vi "Read_FPGA_FIFOs.vi"(6 "TargetB":T1=enum."4", 7 "TargetA":T1, 8 "error in":errorcluster, 9 "#Elements":u32, 11 "FPGA VI Ref":refnum<k20>) -> (0 "error out":errorcluster, 1 "Elements Remaining":u32, 2 "AcqDataB":T2, 3 "AcqDataA":T2)   [LabVIEW 2018]
uses:
  Controls/Clusts/AcqData.ctl
  Controls/Enums/TargetNumber.ctl
  Controls/Clusts/SaturationMonitor.ctl
  Controls/Clusts/FromFPGA_Clust.ctl
  <vilib>/Analysis/baseanly.llb/Mean (DBL).vi
  <vilib>/Utility/error.llb/Error Cluster From Error Code.vi
  <vilib>/rvi/errors/niLvFpgaAdjustHostInterfaceError.vi
  <vilib>/rvi/interface/nirviReadWriteControl/nirviReadWriteControl.xnode
  <vilib>/rvi/interface/nirviMethod/nirviMethod.xnode
  <vilib>/FPGAPlugInAG/Dynamic/niLvFpga_ReadFifo_Dynamic.vi
  <vilib>/rvi/errors/niLvFpgaMergeErrorWithErrorCode.vi
  <vilib>/Analysis/NI_AALBase.lvlib
  NiFpgaLv.dll
  <vilib>/rvi/interface/Simulation/niFpgaSimulationCallBeginRW.vi
panel:
  out "Data":fxp<+/-,24,1>[](array[numeric])
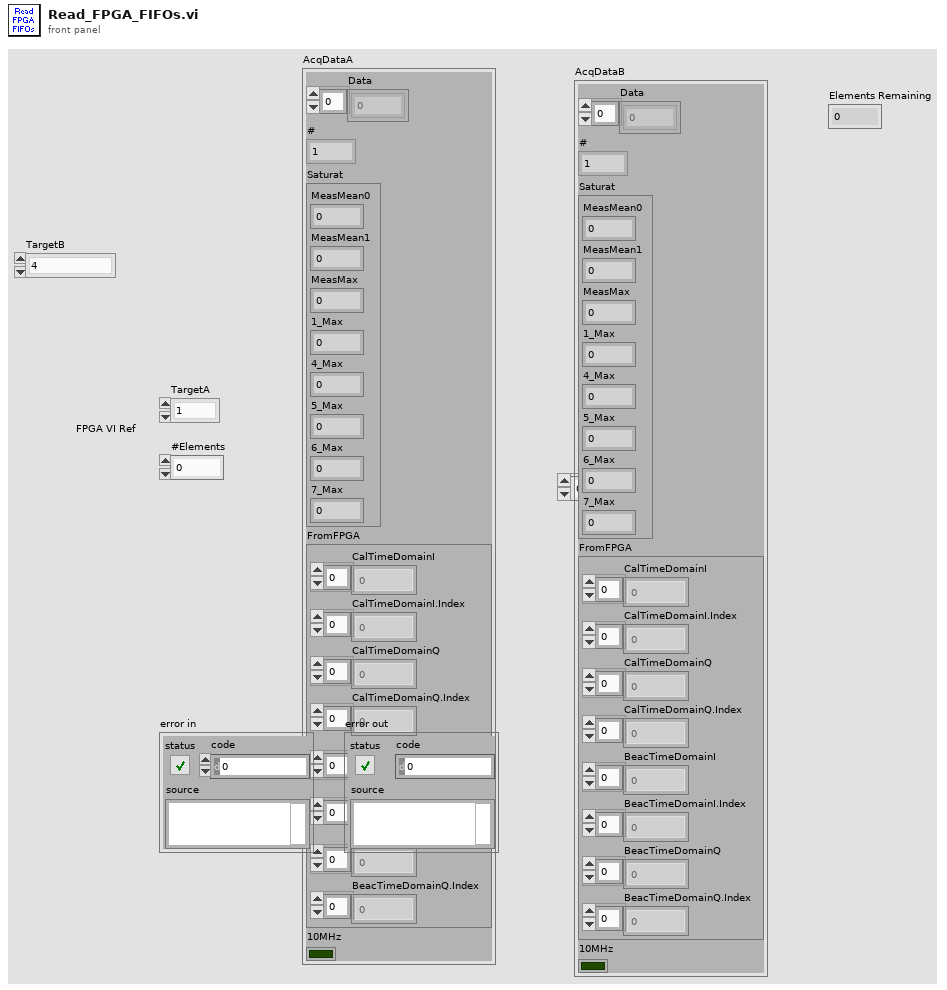
[diagram p1: front panel]
types:
  T1 = typedef "TargetNumber.ctl" = enum16{"1", "2", "3", "4"}
  T2 = typedef "AcqData.ctl" = cluster{"Data":fxp<+/-,24,1>[], "#":T1, "Saturat":T3, "FromFPGA":T4, "10MHz":bool}
  T3 = typedef "SaturationMonitor.ctl" = cluster{"MeasMean0":dbl, "MeasMean1":dbl, "MeasMax":dbl, "1_Max":dbl, "4_Max":dbl, "5_Max":dbl, "6_Max":dbl, "7_Max":dbl}
  T4 = typedef "FromFPGA_Clust.ctl" = cluster{"CalTimeDomainI":ext[], "CalTimeDomainI.Index":ext[], "CalTimeDomainQ":ext[], "CalTimeDomainQ.Index":ext[], "BeacTimeDomainI":ext[], "BeacTimeDomainI.Index":ext[], "BeacTimeDomainQ":ext[], "BeacTimeDomainQ.Index":ext[]}
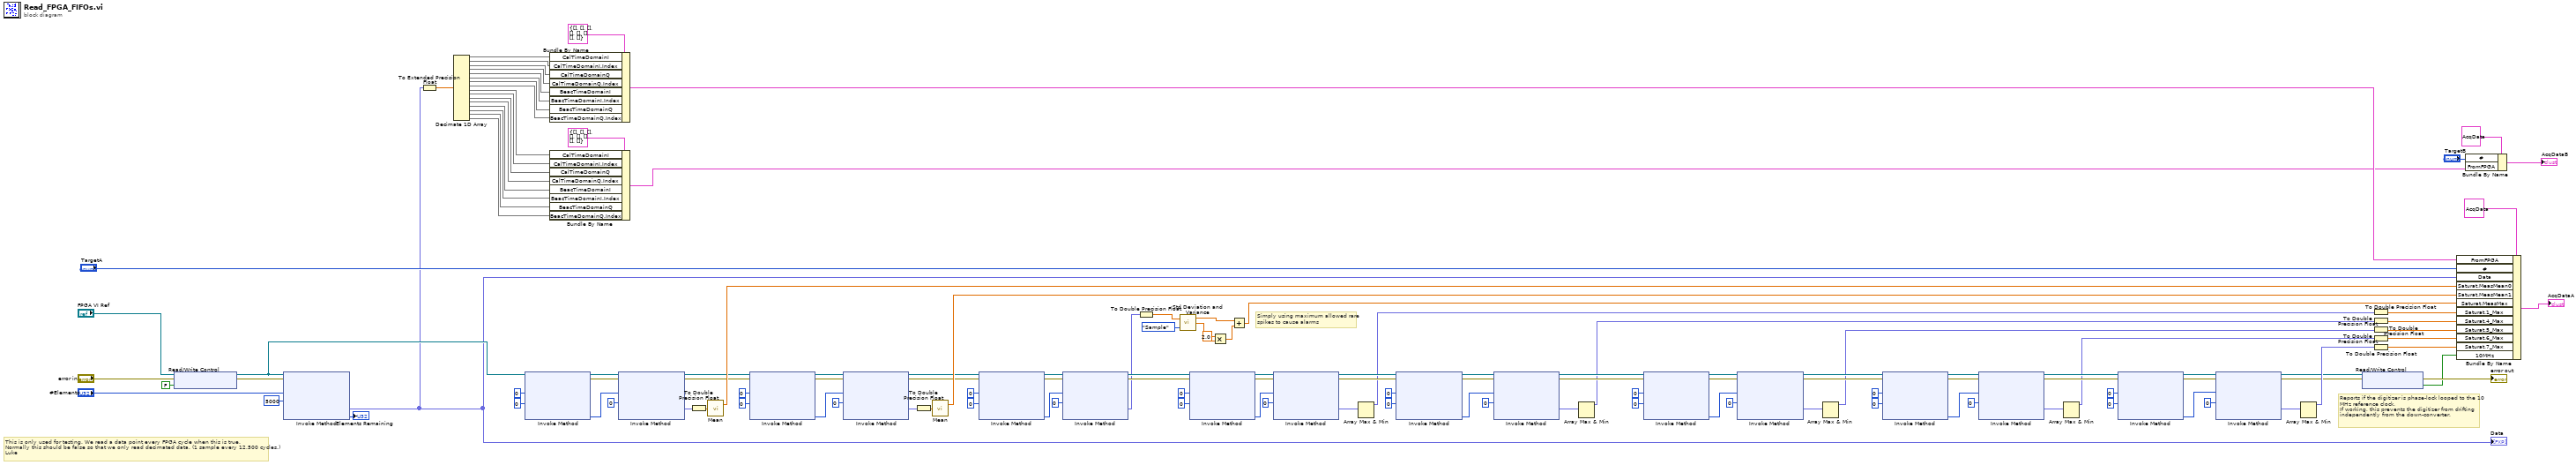
[diagram p0: block diagram]
diagram:
  # "Simply using maximum allowed rare\nspikes to cause alarms"
  # "Reports if the digitizer is phase-lock looped to the 10 MHz reference clock.\nIf working, this prevents the digitizer from drifting independently from the down-converter."
  # "This is only used for testing. We read a data point every FPGA cycle when this is true.\nNormally this should be false so that we only read decimated data. (1 sample every 12,500 cycles.)\nLuke"
  n1 = xnode "Read/Write Control"("FPGA VI Reference In"="FPGA VI Ref", "error in"="error in", "AllData_EvenInvalid"=FALSE ("EnableFIFO")) -> ("FPGA VI Reference Out"=w40:refnum<k20>, "error out"=w41:errorcluster)
  n2 = xnode "Invoke Method"("FPGA VI Reference In"=w40, "error in"=w41, "Number of Elements"="#Elements", "Timeout (ms)"=5000) -> ("Data"=w33:fxp<+/-,24,1>[], "Elements Remaining"=→"Elements Remaining":u32)  [unwired: 2 out]
  "Data" <- w33
  n3 = To Extended Precision Float(1:w33) -> (0:w30:ext[])
  n4 = Decimate 1D Array(w30) -> (w31:ext[], w29:ext[], w28:ext[], w27:ext[], w26:ext[], w25:ext[], w24:ext[], w23:ext[], w22:ext[], w21:ext[], w20:ext[], w19:ext[], w18:ext[], w17:ext[], w16:ext[], w15:ext[])
  n5 = xnode "Invoke Method"("FPGA VI Reference In"=w40, "Number of Elements"=u32 0, "Timeout (ms)"=0) -> ("FPGA VI Reference Out"=w115:refnum<k20>, "error out"=w111:errorcluster, "Elements Remaining"=w112:u32)  [unwired: 1 in, 1 out]
  n6 = Bundle By Name(cluster=T4 {"CalTimeDomainI"=[], "CalTimeDomainI.Index"=[], "CalTimeDomainQ"=[], "CalTimeDomainQ.Index"=[], "BeacTimeDomainI"=[], "BeacTimeDomainI.Index"=[], "BeacTimeDomainQ"=[], "BeacTimeDomainQ.Index"=[]} ("FromFPGA"), "CalTimeDomainI"=w31, "CalTimeDomainI.Index"=w29, "CalTimeDomainQ"=w28, "CalTimeDomainQ.Index"=w27, "BeacTimeDomainI"=w26, "BeacTimeDomainI.Index"=w25, "BeacTimeDomainQ"=w24, "BeacTimeDomainQ.Index"=w23) -> (w14:T4)
  n7 = Bundle By Name(cluster=T4 {"CalTimeDomainI"=[], "CalTimeDomainI.Index"=[], "CalTimeDomainQ"=[], "CalTimeDomainQ.Index"=[], "BeacTimeDomainI"=[], "BeacTimeDomainI.Index"=[], "BeacTimeDomainQ"=[], "BeacTimeDomainQ.Index"=[]} ("FromFPGA"), "CalTimeDomainI"=w22, "CalTimeDomainI.Index"=w21, "CalTimeDomainQ"=w20, "CalTimeDomainQ.Index"=w19, "BeacTimeDomainI"=w18, "BeacTimeDomainI.Index"=w17, "BeacTimeDomainQ"=w16, "BeacTimeDomainQ.Index"=w15) -> (w13:T4)
  n8 = xnode "Invoke Method"("FPGA VI Reference In"=w115, "error in"=w111, "Number of Elements"=w112, "Timeout (ms)"=0) -> ("FPGA VI Reference Out"=w66:refnum<k20>, "error out"=w65:errorcluster, "Data"=w122:fxp<+/-,16,16>[])  [unwired: 1 out]
  n9 = To Double Precision Float(number=w122) -> (double precision float=w123:dbl[])
  n10 = call-poly <vilib>:"Mean.vi"("X"=w123) -> ("mean"=w129:dbl)  [unwired: 1 out]
  n11 = xnode "Invoke Method"("FPGA VI Reference In"=w66, "error in"=w65, "Number of Elements"=u32 0, "Timeout (ms)"=0) -> ("FPGA VI Reference Out"=w70:refnum<k20>, "error out"=w74:errorcluster, "Elements Remaining"=w73:u32)  [unwired: 1 out]
  n12 = xnode "Invoke Method"("FPGA VI Reference In"=w70, "error in"=w74, "Number of Elements"=w73, "Timeout (ms)"=0) -> ("FPGA VI Reference Out"=w47:refnum<k20>, "error out"=w46:errorcluster, "Data"=w68:fxp<+/-,16,16>[])  [unwired: 1 out]
  n13 = To Double Precision Float(number=w68) -> (double precision float=w67:dbl[])
  n14 = call-poly <vilib>:"Mean.vi"("X"=w67) -> ("mean"=w64:dbl)  [unwired: 1 out]
  n15 = xnode "Invoke Method"("FPGA VI Reference In"=w47, "error in"=w46, "Number of Elements"=u32 0, "Timeout (ms)"=0) -> ("FPGA VI Reference Out"=w50:refnum<k20>, "error out"=w49:errorcluster, "Elements Remaining"=w51:u32)  [unwired: 1 out]
  n16 = xnode "Invoke Method"("FPGA VI Reference In"=w50, "error in"=w49, "Number of Elements"=w51, "Timeout (ms)"=0) -> ("FPGA VI Reference Out"=w45:refnum<k20>, "error out"=w44:errorcluster, "Data"=w8:fxp<+/-,16,1>[])  [unwired: 1 out]
  n17 = To Double Precision Float(number=w8) -> (double precision float=w7:dbl[])
  n18 = call <vilib>:"Std Deviation and Variance.vi"("X"=w7, "Weighting (Sample)"=enum16{"Sample", "Population"}."Sample") -> ("mean"=w5:dbl, "standard deviation"=w4:dbl)  [unwired: 1 out]
  n19 = xnode "Invoke Method"("FPGA VI Reference In"=w45, "error in"=w44, "Number of Elements"=u32 0, "Timeout (ms)"=0) -> ("FPGA VI Reference Out"=w109:refnum<k20>, "error out"=w110:errorcluster, "Elements Remaining"=w108:u32)  [unwired: 1 out]
  n20 = Multiply(x=2.0, y=w4) -> (x*y=w2:dbl)
  n21 = Add(x=w5, y=w2) -> (x+y=w1:dbl)
  n22 = xnode "Invoke Method"("FPGA VI Reference In"=w109, "error in"=w110, "Number of Elements"=w108, "Timeout (ms)"=0) -> ("FPGA VI Reference Out"=w104:refnum<k20>, "error out"=w100:errorcluster, "Data"=w79:fxp<+/-,18,1>[])  [unwired: 1 out]
  n23 = Array Max & Min(array=w79) -> (max value=w63:fxp<+/-,18,1>)  [unwired: 3 out]
  n24 = xnode "Invoke Method"("FPGA VI Reference In"=w104, "error in"=w100, "Number of Elements"=u32 0, "Timeout (ms)"=0) -> ("FPGA VI Reference Out"=w105:refnum<k20>, "error out"=w99:errorcluster, "Elements Remaining"=w103:u32)  [unwired: 1 out]
  n25 = xnode "Invoke Method"("FPGA VI Reference In"=w105, "error in"=w99, "Number of Elements"=w103, "Timeout (ms)"=0) -> ("FPGA VI Reference Out"=w98:refnum<k20>, "error out"=w97:errorcluster, "Data"=w78:fxp<+/-,24,1>[])  [unwired: 1 out]
  n26 = Array Max & Min(array=w78) -> (max value=w59:fxp<+/-,24,1>)  [unwired: 3 out]
  n27 = xnode "Invoke Method"("FPGA VI Reference In"=w98, "error in"=w97, "Number of Elements"=u32 0, "Timeout (ms)"=0) -> ("FPGA VI Reference Out"=w95:refnum<k20>, "error out"=w96:errorcluster, "Elements Remaining"=w94:u32)  [unwired: 1 out]
  n28 = xnode "Invoke Method"("FPGA VI Reference In"=w95, "error in"=w96, "Number of Elements"=w94, "Timeout (ms)"=0) -> ("FPGA VI Reference Out"=w90:refnum<k20>, "error out"=w89:errorcluster, "Data"=w77:fxp<+/-,24,1>[])  [unwired: 1 out]
  n29 = Array Max & Min(array=w77) -> (max value=w60:fxp<+/-,24,1>)  [unwired: 3 out]
  n30 = xnode "Invoke Method"("FPGA VI Reference In"=w90, "error in"=w89, "Number of Elements"=u32 0, "Timeout (ms)"=0) -> ("FPGA VI Reference Out"=w91:refnum<k20>, "error out"=w88:errorcluster, "Elements Remaining"=w87:u32)  [unwired: 1 out]
  n31 = xnode "Invoke Method"("FPGA VI Reference In"=w91, "error in"=w88, "Number of Elements"=w87, "Timeout (ms)"=0) -> ("FPGA VI Reference Out"=w83:refnum<k20>, "error out"=w116:errorcluster, "Data"=w76:fxp<+/-,24,1>[])  [unwired: 1 out]
  n32 = Array Max & Min(array=w76) -> (max value=w61:fxp<+/-,24,1>)  [unwired: 3 out]
  n33 = xnode "Invoke Method"("FPGA VI Reference In"=w83, "Number of Elements"=u32 0, "Timeout (ms)"=0) -> ("FPGA VI Reference Out"=w84:refnum<k20>, "Elements Remaining"=w80:u32)  [unwired: 1 in, 2 out]
  n34 = xnode "Invoke Method"("FPGA VI Reference In"=w84, "error in"=w116, "Number of Elements"=w80, "Timeout (ms)"=0) -> ("FPGA VI Reference Out"=w10:refnum<k20>, "error out"=w12:errorcluster, "Data"=w75:fxp<+/-,24,1>[])  [unwired: 1 out]
  n35 = Array Max & Min(array=w75) -> (max value=w62:fxp<+/-,24,1>)  [unwired: 3 out]
  n36 = xnode "Read/Write Control"("FPGA VI Reference In"=w10, "error in"=w12) -> ("error out"=→"error out":errorcluster, "Synthesizer Locked"=w9:bool)  [unwired: 1 out]
  n37 = To Double Precision Float(number=w63) -> (double precision float=w58:dbl)
  n38 = To Double Precision Float(number=w59) -> (double precision float=w57:dbl)
  n39 = To Double Precision Float(number=w60) -> (double precision float=w56:dbl)
  n40 = To Double Precision Float(number=w61) -> (double precision float=w55:dbl)
  n41 = To Double Precision Float(number=w62) -> (double precision float=w54:dbl)
  n42 = Bundle By Name(cluster=T2 {"Data"=[], "#"=enum."1", "Saturat"={"MeasMean0"=0.0, "MeasMean1"=0.0, "MeasMax"=0.0, "1_Max"=0.0, "4_Max"=0.0, "5_Max"=0.0, "6_Max"=0.0, "7_Max"=0.0}, "FromFPGA"={"CalTimeDomainI"=[], "CalTimeDomainI.Index"=[], "CalTimeDomainQ"=[], "CalTimeDomainQ.Index"=[], "BeacTimeDomainI"=[], "BeacTimeDomainI.Index"=[], "BeacTimeDomainQ"=[], "BeacTimeDomainQ.Index"=[]}, "10MHz"=FALSE}, "FromFPGA"=w14, "#"="TargetA", "Data"=w33, "Saturat.MeasMean0"=w129, "Saturat.MeasMean1"=w64, "Saturat.MeasMax"=w1, "Saturat.1_Max"=w58, "Saturat.4_Max"=w57, "Saturat.5_Max"=w56, "Saturat.6_Max"=w55, "Saturat.7_Max"=w54, "10MHz"=w9) -> (→"AcqDataA":T2)
  n43 = Bundle By Name(cluster=T2 {"Data"=[], "#"=enum."1", "Saturat"={"MeasMean0"=0.0, "MeasMean1"=0.0, "MeasMax"=0.0, "1_Max"=0.0, "4_Max"=0.0, "5_Max"=0.0, "6_Max"=0.0, "7_Max"=0.0}, "FromFPGA"={"CalTimeDomainI"=[], "CalTimeDomainI.Index"=[], "CalTimeDomainQ"=[], "CalTimeDomainQ.Index"=[], "BeacTimeDomainI"=[], "BeacTimeDomainI.Index"=[], "BeacTimeDomainQ"=[], "BeacTimeDomainQ.Index"=[]}, "10MHz"=FALSE}, "#"="TargetB", "FromFPGA"=w13) -> (→"AcqDataB":T2)
